vi "Tektronix DPO MSO 2000 4000 Series Create Standard Waveforms Example.vi"() -> ()   [LabVIEW 2016]
doc: "This example illustrates how to configure and output a standard waveform.\n\n<B>Notes:</B>\n(1) This VI is available for MDO3000 Series only.\n\n(2) Requires the MDO3AFG option to be installed."
uses:
  <instrlib>/Tektronix DPO MSO 2000 4000 Series/Tektronix DPO MSO 2000 4000 Series.lvlib
panel:
  in  "VISA Resource Name":refnum<visa-resource-name>
  in  "DC Offset (0 V)":dbl
  in  "Amplitude (0.5 V)":dbl=0.5
  in  "Waveform Function (0: Sine)":i32(ring) items=["Sine", "Square", "Pulse", "Ramp", "Noise", "DC", "Sinc", "Gaussian", "Lorentz", "Exponential Rise", "Exponential Decay", "Haversine", "Cardiac"]
  in  "Impedance (1: High Impedance)":i32(ring)=1 items=["50 Ohms", "High Impedance"]
  # "(C)2006 - 2016. National Instruments Corporation. ALL RIGHTS RESERVED."
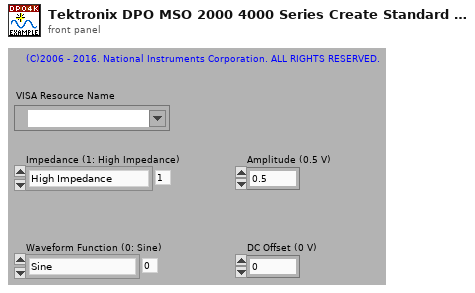
[diagram p1: front panel]
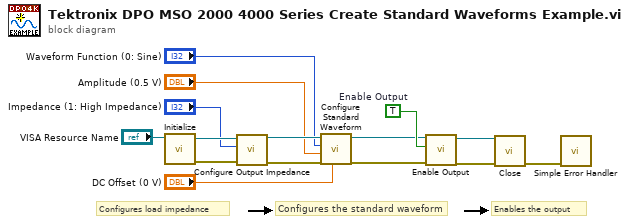
[diagram p0: block diagram]
diagram:
  w9 = TRUE  # Enable Output
  # "Enables the output"
  # "Configures the standard waveform"
  # "Configures load impedance"
  n1 = call <instrlib>:"Initialize.vi"("VISA resource name"="VISA Resource Name") -> ("error out"=w13:errorcluster, "VISA resource name out"=w14:refnum<visa-resource-name>)  [unwired: 9 in]
  n2 = call <instrlib>:"Configure Output Impedance.vi"("error in (no error)"=w13, "Impedance (1: High Impedance)"="Impedance (1: High Impedance)", "VISA resource name"=w14) -> ("error out"=w7:errorcluster, "VISA resource name out"=w8:refnum<visa-resource-name>)  [unwired: 7 in]
  n3 = call <instrlib>:"Configure Standard Waveform.vi"("DC Offset (0 V)"="DC Offset (0 V)", "error in (no error)"=w7, "Amplitude (0.5 V)"="Amplitude (0.5 V)", "Waveform Function (0: Sine)"="Waveform Function (0: Sine)", "VISA resource name"=w8) -> ("error out"=w5:errorcluster, "VISA resource name out"=w6:refnum<visa-resource-name>)  [unwired: 5 in]
  n4 = call <instrlib>:"Enable Output.vi"("error in (no error)"=w5, "Enable Output (F: Disable)"=w9, "VISA resource name"=w6) -> ("error out"=w11:errorcluster, "VISA resource name out"=w12:refnum<visa-resource-name>)  [unwired: 7 in]
  n5 = call <instrlib>:"Close.vi"("error in (no error)"=w11, "VISA resource name"=w12) -> ("error out"=w15:errorcluster)  [unwired: 9 in]
  n6 = call <vilib>:"Simple Error Handler.vi"("error in (no error)"=w15) -> ()  [unwired: 4 in, 5 out]
